vi "读取DBL_A.vi"(8 "error in (no error)":errorcluster caption="错误输入（无错误）", 11 "运算类输入":refnum<class "运算类.lvclass">) -> (0 "error out":errorcluster caption="错误输出", 2 "DBL_A":dbl, 3 "运算类输出":refnum<class "运算类.lvclass">)   [LabVIEW 2013, in "运算类.lvclass"]
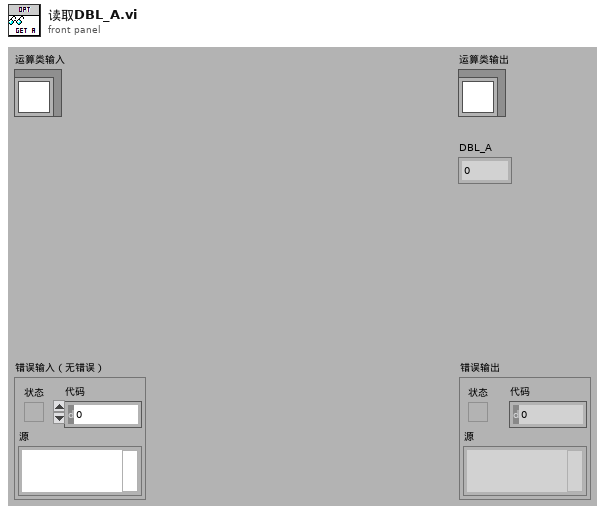
[diagram p1: front panel]
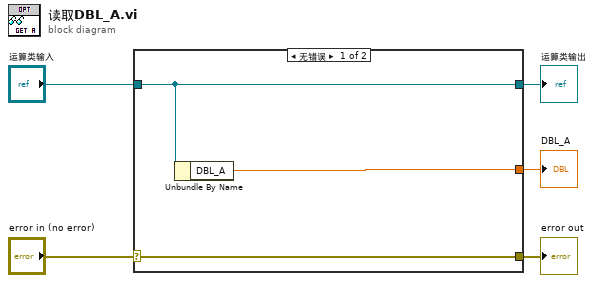
[diagram p0: block diagram]
diagram:
  n1 = case shown="无错误" "error in (no error)" {
    selector: "error in (no error)" -> [w8 w9]
    tunnel: [w8 w9] -> w4
    tunnel: [w7 w10] -> w2
    tunnel: "运算类输入" -> [w7 w10]
    tunnel: [w6 _] -> w1
    frame No Error {
      n2 = Unbundle By Name(w7) -> ("DBL_A"=w6:dbl)
    }
    frame Error {
    }
  }
  "error out" <- w4
  "运算类输出" <- w2
  "DBL_A" <- w1
